vi "somma roi.vi"(9 "ROIs Min Max":i32[][](array[numeric]), 11 "Data loaded reference In":refnum<data-value>) -> (1 "ROIs Array Out":i32[][](array[numeric]))   [LabVIEW 2023]
panel:
  out "element 2":i32
  out "element":i32
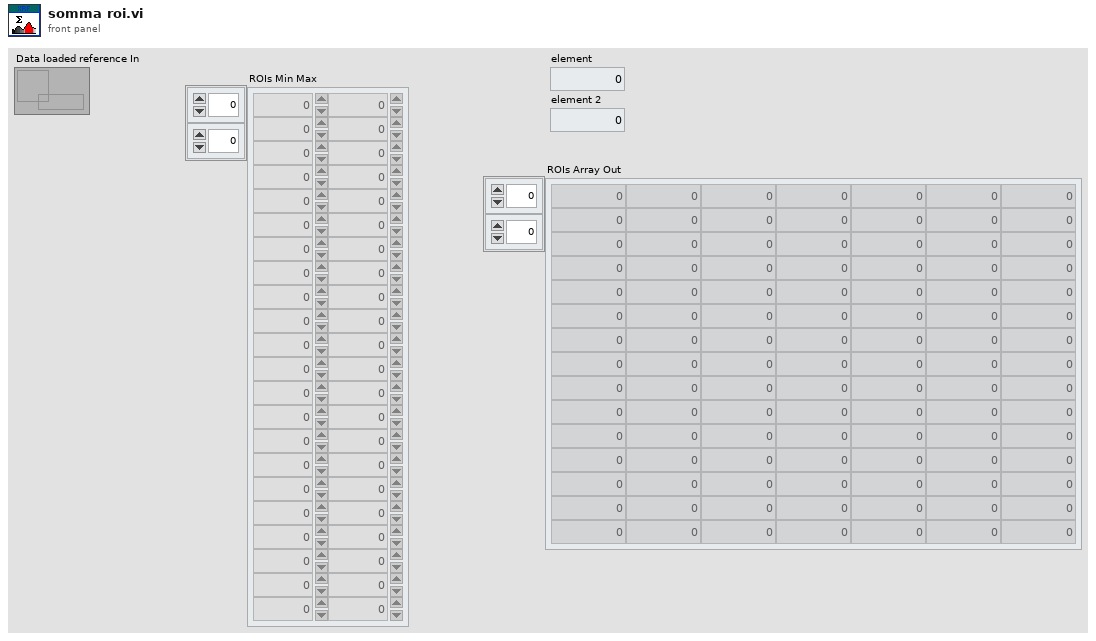
[diagram p1: front panel]
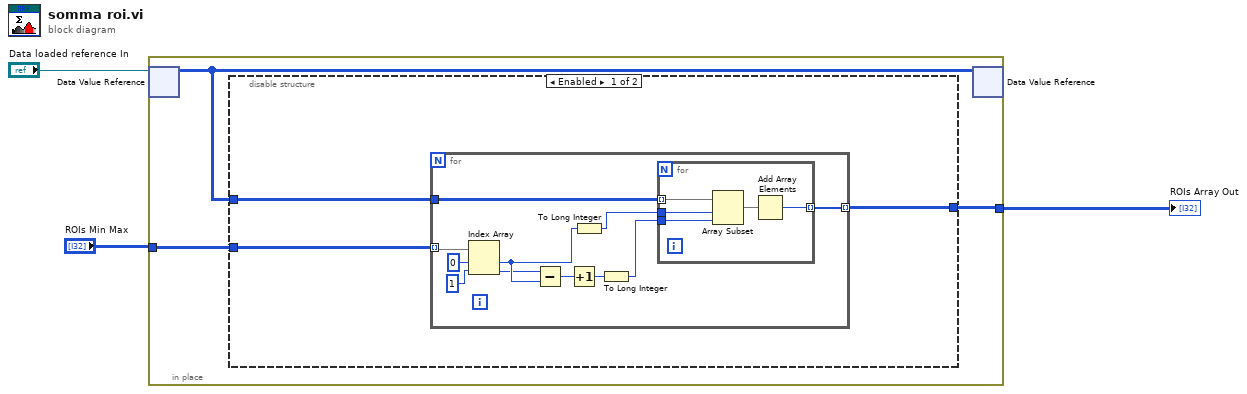
[diagram p0: block diagram]
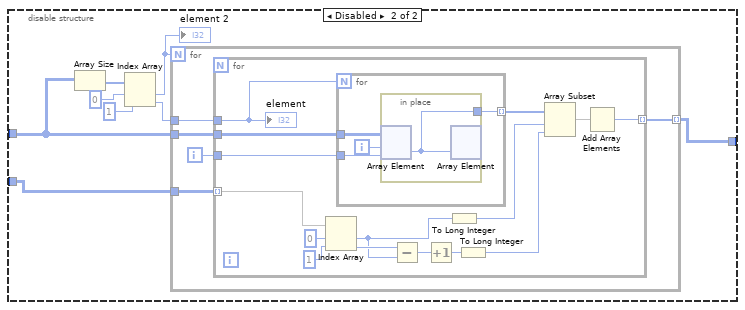
[diagram p2: hidden frame]
diagram:
  n1 = in-place {
    in-place-border: "ROIs Min Max" -> [w6]
    in-place-border: [w5] -> w2
    n2 = in-place-dvr #1("Data loaded reference In") -> (w4:i32[][])  [unwired: 1 out]
    n3 = disable-structure shown="Enabled" {
      disable-tunnel: w6 -> [w9 w27]
      disable-tunnel: [w8 w26] -> w5
      disable-tunnel: w4 -> [w7 w28]
      frame Enabled {
        n4 = for {
          tunnel: w9 -> [w20] mode=indexing
          tunnel: w7 -> [w11]
          tunnel: [w10] -> w8 mode=indexing
          n5 = Index Array(array=w20, index #1=0 ("index"), index #2=1 ("index")) -> (element #1=w15:i32, element #2=w14:i32)
          n6 = Subtract(x=w14, y=w15) -> (x-y=w17:i32)
          n7 = Increment(x=w17) -> (x+1=w16:i32)
          n8 = To Long Integer(number=w15) -> (32bit integer=w13:i32)
          n9 = To Long Integer(number=w16) -> (32bit integer=w12:i32)
          n10 = for {
            tunnel: w13 -> [w25]
            tunnel: w12 -> [w24]
            tunnel: w11 -> [w22] mode=indexing
            tunnel: [w21] -> w10 mode=indexing
            n11 = Array Subset(array=w22, index=w25, length=w24) -> (w23:i32[])
            n12 = Add Array Elements(numeric array=w23) -> (sum=w21:i32)
          }
        }
      }
      frame Disabled {
        n13 = Array Size(array=w28) -> (size(s)=w31:i32[])
        n14 = Index Array(array=w31, index #1=0 ("index"), index #2=1 ("index")) -> (element #1=w32:i32, element #2=w33:i32)
        "element 2" <- w32
        n15 = for {
          N: w32 -> [_]
          tunnel: w28 -> [w35]
          tunnel: w27 -> [w37]
          tunnel: [w36] -> w26 mode=indexing
          tunnel: w33 -> [w34]
          i -> [w38]
          n16 = for {
            tunnel: w38 -> [w53]
            tunnel: w37 -> [w46] mode=indexing
            tunnel: [w43] -> w36 mode=indexing
            tunnel: w35 -> [w40]
            tunnel: w34 -> [w39]
            n17 = Index Array(array=w46, index #1=0 ("index"), index #2=1 ("index")) -> (element #1=w51:i32, element #2=w52:i32)
            n18 = for {
              N: w39 -> [_]
              tunnel: w40 -> [w57]
              tunnel: w53 -> [w55]
              tunnel: [w54] -> w44 mode=indexing
              i -> [w56]
              n19 = in-place {
                in-place-border: [w58] -> w54
                n20 = in-place-array #2(w57, w56, w55) -> (w58:i32)
                n21 = in-place-array #2(w58) -> ()  [unwired: 3 out]
              }
            }
            n22 = Subtract(x=w52, y=w51) -> (x-y=w49:i32)
            n23 = Increment(x=w49) -> (x+1=w50:i32)
            n24 = To Long Integer(number=w51) -> (32bit integer=w42:i32)
            n25 = To Long Integer(number=w50) -> (32bit integer=w41:i32)
            n26 = Array Subset(array=w44, index=w42, length=w41) -> (w45:i32[])
            n27 = Add Array Elements(numeric array=w45) -> (sum=w43:i32)
            "element" <- w39
          }
        }
      }
    }
    n28 = in-place-dvr #1(w4) -> ()  [unwired: 2 out]
  }
  "ROIs Array Out" <- w2
